vi "-8730 Attribute not found--error.vi"(8 "error in":errorcluster, 11 "Attribute":string) -> (0 "error out":errorcluster)   [LabVIEW 2024, in "PCAN.lvlib" / "Config Hardcoded.lvclass"]
uses:
  Config Hardcoded.lvclass
  Config Hardcoded.lvclass/Config Hardcoded.ctl
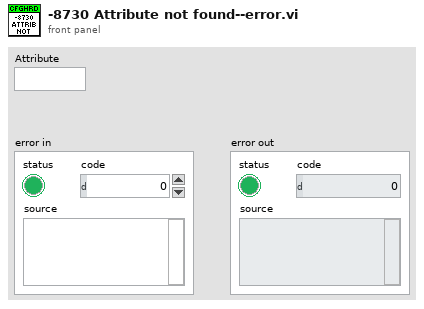
[diagram p1: front panel]
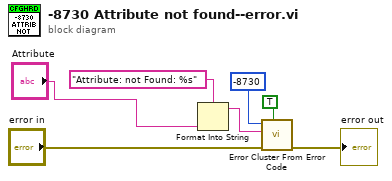
[diagram p0: block diagram]
diagram:
  n1 = Format Into String(format string="Attribute: not Found: %s" ("error message (\"\")"), "Attribute") -> (resulting string=w5:string)  [unwired: 2 in, 1 out]
  n2 = call <vilib>:"Error Cluster From Error Code.vi"("show call chain? (False)"=TRUE, "error in (no error)"="error in", "error message (\"\")"=w5, "error code (0)"=-8730) -> ("error out"=→"error out":errorcluster)  [unwired: 5 in]
